vi "Str2Str(remove ascii).vi"(1 "string":string) -> (0 "string sql":string)   [LabVIEW 2019, in "Tools.lvlib"]
uses:
  Tools.lvlib
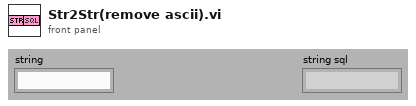
[diagram p1: front panel]
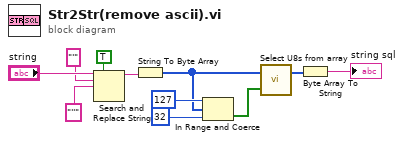
[diagram p0: block diagram]
diagram:
  n1 = Search and Replace String(replace all?=TRUE ("replace all? (F)"), input string="string", search string="'", replace string="''") -> (result string=w8:string)  [unwired: 4 in, 3 out]
  n2 = String To Byte Array(string=w8) -> (unsigned byte array=w5:u8[])
  n3 = In Range and Coerce(upper limit=u8 127, x=w5, lower limit=u8 32) -> (In Range?=w3:bool[])  [unwired: 1 out]
  n4 = call "Select U8s from array.vi"("selection array"=w3, "I32s"=w5) -> ("selected I32s"=w7:u8[])  [unwired: 1 in]
  n5 = Byte Array To String(unsigned byte array=w7) -> (string=→"string sql":string)
